vi "_builtins_rect_align.vi"(10 "Align Type":T2, 11 "Rects in":T1[](array[typedef])) -> (3 "Resolved Rects out":T1[](array[typedef]))   [LabVIEW 2019, in "Script.lvlib"]
doc: "Calculates the relative move for the selected alignment using the Master Bound Rectangles (excludes labels, captions, and display objects).\n\nCreated by: Ryan Pacini"
uses:
  Script.lvlib
  _builtins_align.ctl
  <vilib>/Utility/miscctls.llb/LVRectTypeDef.ctl
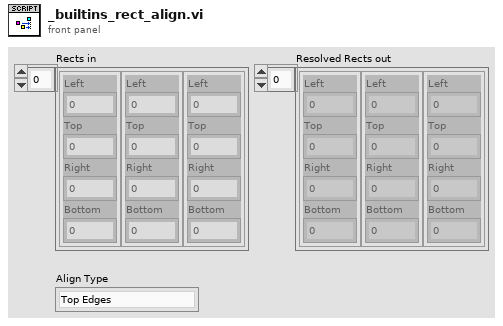
[diagram p1: front panel]
types:
  T1 = typedef "LVRectTypeDef.ctl" = cluster{"Left":i16, "Top":i16, "Right":i16, "Bottom":i16}
  T2 = typedef "Script.lvlib/_builtins_align.ctl" = enum8{"Top Edges", "Vertical Centers", "Bottom Edges", "Left Edges", "Horizontal Centers", "Right Edges"}
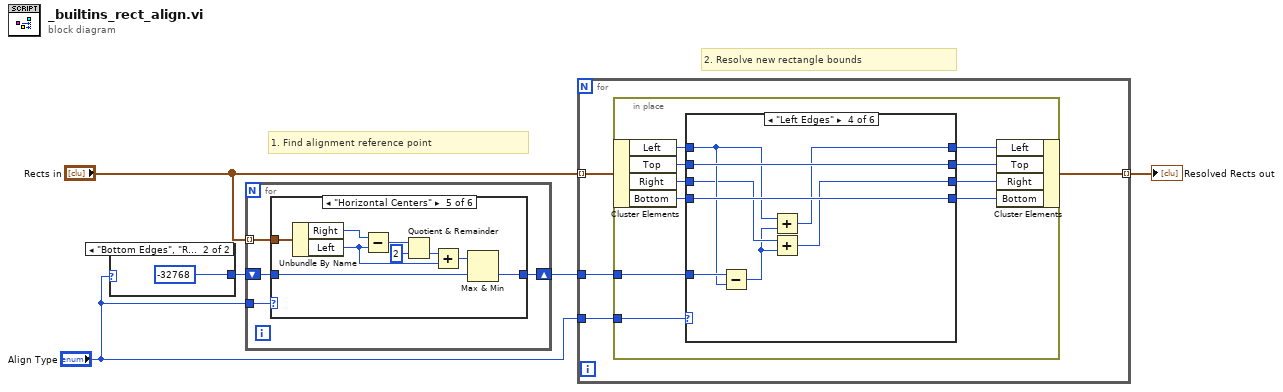
[diagram p0: block diagram]
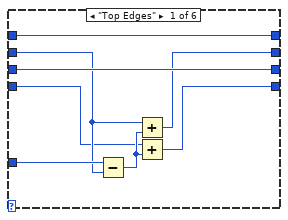
[diagram p2: hidden frame]
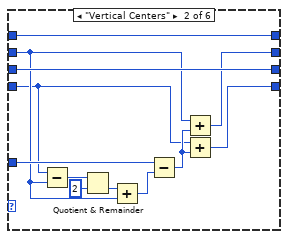
[diagram p3: hidden frame]
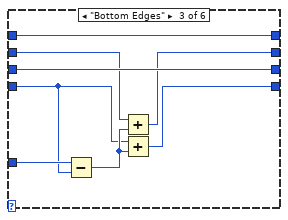
[diagram p4: hidden frame]
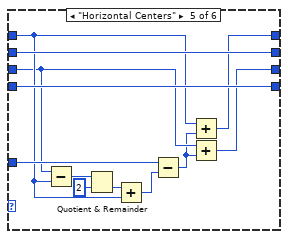
[diagram p5: hidden frame]
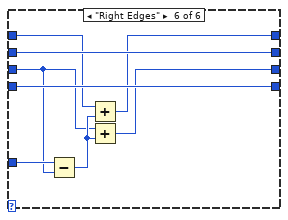
[diagram p6: hidden frame]
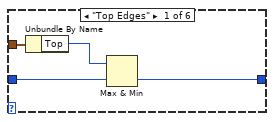
[diagram p7: hidden frame]
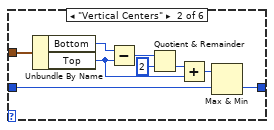
[diagram p8: hidden frame]
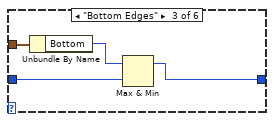
[diagram p9: hidden frame]
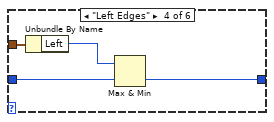
[diagram p10: hidden frame]
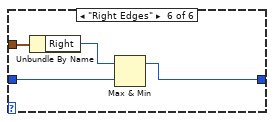
[diagram p11: hidden frame]
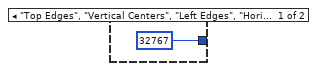
[diagram p12: hidden frame]
diagram:
  # "2. Resolve new rectangle bounds"
  # "1. Find alignment reference point"
  n1 = case shown="\"Bottom Edges\", \"Right Edges\"" "Align Type" {
    tunnel: [i16 32767 ("Left") i16 -32768 ("Left")] -> w3
    frame "Top Edges", "Vertical Centers", "Left Edges", "Horizontal Centers" {
    }
    frame "Bottom Edges", "Right Edges" {
    }
  }
  n2 = for {
    tunnel: "Align Type" -> [w11]
    shift-right: [w9] -> w4
    shift-left: w3 -> [w10]
    tunnel: "Rects in" -> [w8] mode=indexing
    n3 = case shown="\"Horizontal Centers\"" w11 {
      tunnel: w8 -> [w14 w22 w27 w30 w39 w44]
      tunnel: w10 -> [w15 w24 w28 w32 w41 w45]
      tunnel: [w12 w23 w25 w31 w40 w42] -> w9
      frame "Top Edges" {
        n4 = Unbundle By Name(w14) -> ("Top"=w13:i16)
        n5 = Max & Min(x=w13, y=w15) -> (min(x,y)=w12:i16)  [unwired: 1 out]
      }
      frame "Vertical Centers" {
        n6 = Unbundle By Name(w22) -> ("Bottom"=w21:i16, "Top"=w17:i16)
        n7 = Subtract(x=w21, y=w17) -> (x-y=w20:i16)
        n8 = Quotient & Remainder(x=w20, y=i16 2) -> (floor(x/y)=w18:i16)  [unwired: 1 out]
        n9 = Add(x=w18, y=w17) -> (x+y=w16:i16)
        n10 = Max & Min(x=w16, y=w24) -> (min(x,y)=w23:i16)  [unwired: 1 out]
      }
      frame "Bottom Edges" {
        n11 = Unbundle By Name(w27) -> ("Bottom"=w26:i16)
        n12 = Max & Min(x=w26, y=w28) -> (max(x,y)=w25:i16)  [unwired: 1 out]
      }
      frame "Left Edges" {
        n13 = Unbundle By Name(w30) -> ("Left"=w29:i16)
        n14 = Max & Min(x=w29, y=w32) -> (min(x,y)=w31:i16)  [unwired: 1 out]
      }
      frame "Horizontal Centers" {
        n15 = Unbundle By Name(w39) -> ("Right"=w38:i16, "Left"=w34:i16)
        n16 = Subtract(x=w38, y=w34) -> (x-y=w37:i16)
        n17 = Quotient & Remainder(x=w37, y=i16 2) -> (floor(x/y)=w35:i16)  [unwired: 1 out]
        n18 = Add(x=w35, y=w34) -> (x+y=w33:i16)
        n19 = Max & Min(x=w33, y=w41) -> (min(x,y)=w40:i16)  [unwired: 1 out]
      }
      frame "Right Edges" {
        n20 = Unbundle By Name(w44) -> ("Right"=w43:i16)
        n21 = Max & Min(x=w43, y=w45) -> (max(x,y)=w42:i16)  [unwired: 1 out]
      }
    }
  }
  n22 = for {
    tunnel: w4 -> [w49]
    tunnel: "Rects in" -> [w47] mode=indexing
    tunnel: "Align Type" -> [w48]
    tunnel: [w46] -> w1 mode=indexing
    n23 = in-place {
      in-place-border: w49 -> [w59]
      in-place-border: w48 -> [w58]
      n24 = in-place-cluster #1(w47) -> ("Left"=w56:i16, "Top"=w54:i16, "Right"=w52:i16, "Bottom"=w50:i16)
      n25 = case shown="\"Left Edges\"" w58 {
        tunnel: w59 -> [w67 w79 w87 w95 w107 w115]
        tunnel: [w66 w74 w86 w92 w100 w111] -> w57
        tunnel: w56 -> [w66 w74 w86 w91 w99 w110]
        tunnel: [w64 w71 w83 w94 w102 w114] -> w55
        tunnel: w54 -> [w63 w70 w82 w94 w102 w114]
        tunnel: [w65 w73 w85 w90 w98 w109] -> w53
        tunnel: w52 -> [w65 w73 w85 w89 w97 w108]
        tunnel: [w61 w69 w81 w93 w101 w113] -> w51
        tunnel: w50 -> [w60 w68 w80 w93 w101 w113]
        frame "Top Edges" {
          n26 = Subtract(x=w67, y=w63) -> (x-y=w62:i16)
          n27 = Add(x=w63, y=w62) -> (x+y=w64:i16)
          n28 = Add(x=w60, y=w62) -> (x+y=w61:i16)
        }
        frame "Vertical Centers" {
          n29 = Subtract(x=w68, y=w70) -> (x-y=w78:i16)
          n30 = Quotient & Remainder(x=w78, y=i16 2) -> (floor(x/y)=w76:i16)  [unwired: 1 out]
          n31 = Add(x=w76, y=w70) -> (x+y=w75:i16)
          n32 = Subtract(x=w79, y=w75) -> (x-y=w72:i16)
          n33 = Add(x=w70, y=w72) -> (x+y=w71:i16)
          n34 = Add(x=w68, y=w72) -> (x+y=w69:i16)
        }
        frame "Bottom Edges" {
          n35 = Subtract(x=w87, y=w80) -> (x-y=w84:i16)
          n36 = Add(x=w82, y=w84) -> (x+y=w83:i16)
          n37 = Add(x=w80, y=w84) -> (x+y=w81:i16)
        }
        frame "Left Edges" {
          n38 = Subtract(x=w95, y=w91) -> (x-y=w88:i16)
          n39 = Add(x=w91, y=w88) -> (x+y=w92:i16)
          n40 = Add(x=w89, y=w88) -> (x+y=w90:i16)
        }
        frame "Horizontal Centers" {
          n41 = Subtract(x=w97, y=w99) -> (x-y=w106:i16)
          n42 = Quotient & Remainder(x=w106, y=i16 2) -> (floor(x/y)=w104:i16)  [unwired: 1 out]
          n43 = Add(x=w104, y=w99) -> (x+y=w103:i16)
          n44 = Subtract(x=w107, y=w103) -> (x-y=w96:i16)
          n45 = Add(x=w99, y=w96) -> (x+y=w100:i16)
          n46 = Add(x=w97, y=w96) -> (x+y=w98:i16)
        }
        frame "Right Edges" {
          n47 = Subtract(x=w115, y=w108) -> (x-y=w112:i16)
          n48 = Add(x=w110, y=w112) -> (x+y=w111:i16)
          n49 = Add(x=w108, y=w112) -> (x+y=w109:i16)
        }
      }
      n50 = in-place-cluster #1("Left"=w57, "Top"=w55, "Right"=w53, "Bottom"=w51) -> (w46:T1)
    }
  }
  "Resolved Rects out" <- w1
